vi "Atheros xtal CAL INIT.vi"(4 "XtalCalOtpSaveOption":u32, 6 "XtalCapDelta":i32, 8 "error in (no error)":errorcluster, 9 "XtalTolerancePPM":u32, 10 "XtalTargetPPM":i32, 11 "_hResourceContext":u32) -> (0 "error out":errorcluster, 2 "function return":bool, 3 "_hResourceContext out":u32)   [LabVIEW 2013, in "QCAWLAN_DLL.lvlib"]
doc: "QCA_DLL_Export bool Atheros_xtal_CAL_INIT (HANDLE _hResourceContext, int XtalTargetPPM, unsigned int XtalTolerancePPM, int XtalCapDelta, unsigned XtalCalOtpSaveOption);"
uses:
  QCAWLAN_DLL.lvlib
  QCAWLAN_DLL.dll
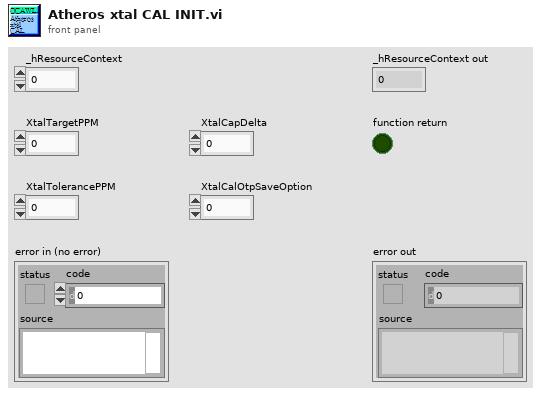
[diagram p1: front panel]
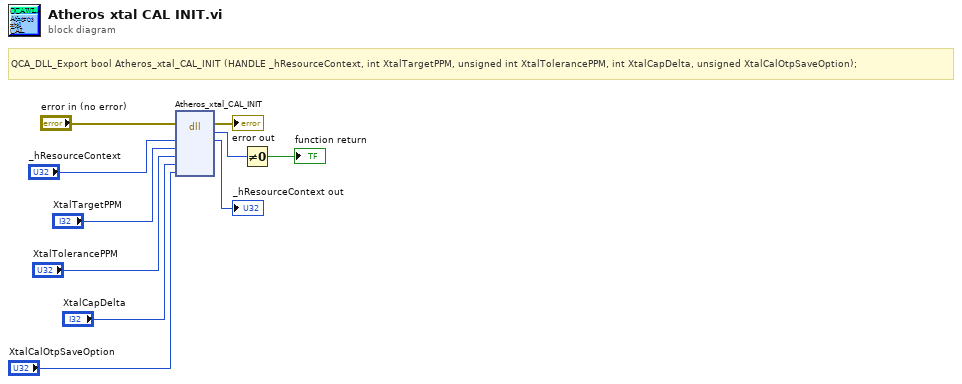
[diagram p0: block diagram]
diagram:
  # "QCA_DLL_Export bool Atheros_xtal_CAL_INIT (HANDLE _hResourceContext, int XtalTargetPPM, unsigned int XtalTolerancePPM, int XtalCapDelta, unsigned XtalCalOtpSaveOption);"
  n1 = dll-call lib="C:/Connectivity Client - MIMO/PlugIn/QCAWLAN_DLL.*" fn="Atheros_xtal_CAL_INIT"(error in="error in (no error)", "_hResourceContext"="_hResourceContext", "XtalTargetPPM"="XtalTargetPPM", "XtalTolerancePPM"="XtalTolerancePPM", "XtalCapDelta"="XtalCapDelta", "XtalCalOtpSaveOption"="XtalCalOtpSaveOption") -> (error out=→"error out":errorcluster, w9:u8, "_hResourceContext"=→"_hResourceContext out":u32)  [unwired: 6 in, 1 out]
  n2 = Not Equal To 0?(x=w9) -> (x != 0?=→"function return":bool)
